vi "Set Cluster as Properties.vi"(8 "error in":errorcluster, 10 "Variant Cluster":variant, 11 "custom device ref in":T1 format="%.0x") -> (0 "error out":errorcluster, 3 "custom device ref out":T1 format="%.0x")   [LabVIEW 2020, in "AIM ARINC 664 Scripting.lvlib"]
uses:
  AIM ARINC 664 Scripting.lvlib
  <vilib>/NI VeriStand/Custom Device API/Custom Device Item Ref.ctl
  <vilib>/NI VeriStand/Custom Device API/Set Item Property (U32).vi
  <vilib>/NI VeriStand/Custom Device API/Set Item Property (Boolean).vi
  <vilib>/NI VeriStand/Custom Device API/Set Item Property (String).vi
  <vilib>/NI VeriStand/Custom Device API/Set Item Property (Path).vi
  <vilib>/NI VeriStand/Custom Device API/Custom Device API.lvlib
  <vilib>/Utility/Data Type/NI_Data Type.lvlib
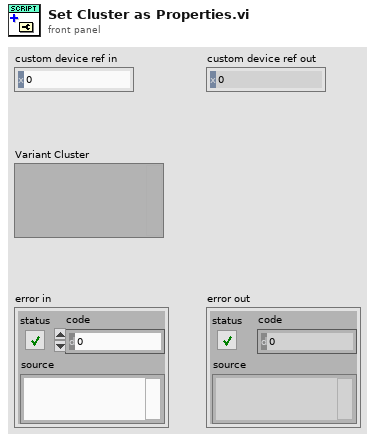
[diagram p1: front panel]
types:
  T1 = typedef "Custom Device API.lvlib/Custom Device Item Ref.ctl" = u64
  T2 = typedef "NI_Data Type.lvlib/Data Type.ctl" = enum8{"Invalid Type", "Void", "I8", "I16", "I32", "I64", "U8", "U16", "U32", "U64", "Single Float", "Double Float", "Extended Float", "Single Complex", "Double Complex", "Extended Complex", "Enum U8", "Enum U16", "Enum U32", "Enum U64", "Single Float With Unit", "Double Float With Unit", "Extended Float With Unit", "Single Complex with Unit", "Double Complex with Unit", "Extended Complex with Unit", "Boolean", "String", "Path", "Picture", "Tag", "Array", "Cluster", "Variant", "LV Variant", "Waveform", "Timestamp", "Digital Waveform", "Digital Data", "ExpressData", "Refnum", "External Data", "VI", "Poly VI", "LabVIEW Class Instance", "Fixed Point", "Set Collection", "Map Collection"}
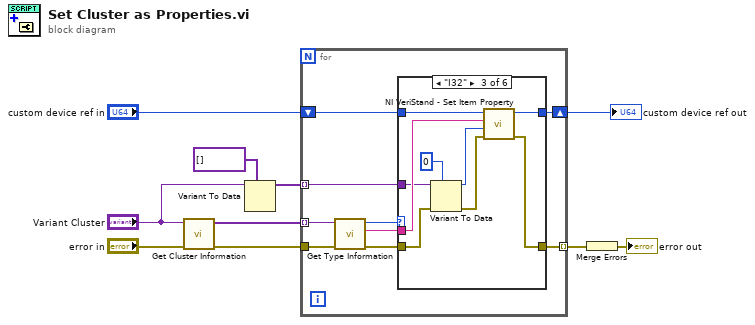
[diagram p0: block diagram]
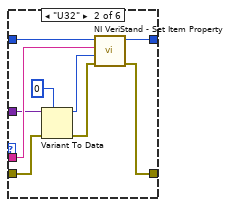
[diagram p3: hidden frame]
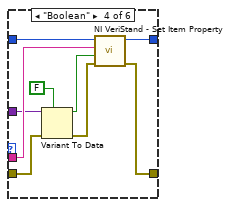
[diagram p4: hidden frame]
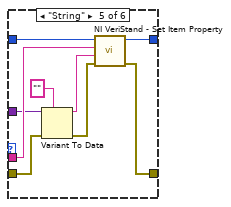
[diagram p5: hidden frame]
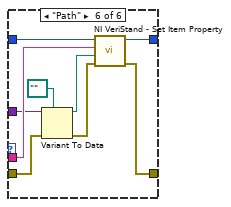
[diagram p6: hidden frame]
diagram:
  n1 = call <vilib>:"Get Cluster Information.vi"("error in (no error)"="error in", "variant"="Variant Cluster") -> ("error out"=w5:errorcluster, "cluster elements"=w6:variant[])  [unwired: 8 in]
  n2 = Variant To Data(type=variant[] [], Variant="Variant Cluster") -> (data=w4:variant[])  [unwired: 1 in, 1 out]
  n3 = for {
    tunnel: w6 -> [w19] mode=indexing
    shift-right: [w15] -> w8
    shift-left: "custom device ref in" -> [w16]
    tunnel: w4 -> [w11] mode=indexing
    tunnel: w5 -> [w18]
    tunnel: [w12] -> w9 mode=indexing
    n4 = call <vilib>:"Get Type Information.vi"("error in (no error)"=w18, "variant"=w19) -> ("error out"=w13:errorcluster, "name"=w17:string, "type"=w14:T2)  [unwired: 5 in, 2 out]
    n5 = case shown="\"I32\"" w14 {
      tunnel: w17 -> [_ w30 w39 w48 w57 w66]
      tunnel: w16 -> [w21 w29 w38 w47 w56 w65]
      tunnel: [w21 w28 w37 w46 w55 w64] -> w15
      tunnel: w13 -> [w20 w23 w32 w41 w50 w59]
      tunnel: [w20 w27 w36 w45 w54 w63] -> w12
      tunnel: w11 -> [_ w26 w35 w44 w53 w62]
      frame "Invalid Type", Default {
      }
      frame "U32" {
        n6 = Variant To Data(error in=w23, type=u32 0, Variant=w26) -> (data=w25:u32, error out=w22:errorcluster)
        n7 = call-poly <vilib>:"NI VeriStand - Set Item Property.vi"("error in (no error)"=w22, "Value"=w25, "Property Name"=w30, "Item Ref in"=w29) -> ("error out"=w27:errorcluster, "Item Ref out"=w28:T1)  [unwired: 5 in, 1 out]
      }
      frame "I32" {
        n8 = Variant To Data(error in=w32, type=0, Variant=w35) -> (data=w34:i32, error out=w31:errorcluster)
        n9 = call-poly <vilib>:"NI VeriStand - Set Item Property.vi"("error in (no error)"=w31, "Value"=w34, "Property Name"=w39, "Item Ref in"=w38) -> ("error out"=w36:errorcluster, "Item Ref out"=w37:T1)  [unwired: 5 in, 1 out]
      }
      frame "Boolean" {
        n10 = Variant To Data(error in=w41, type=FALSE, Variant=w44) -> (data=w43:bool, error out=w40:errorcluster)
        n11 = call-poly <vilib>:"NI VeriStand - Set Item Property.vi"("error in (no error)"=w40, "Value"=w43, "Property Name"=w48, "Item Ref in"=w47) -> ("error out"=w45:errorcluster, "Item Ref out"=w46:T1)  [unwired: 5 in, 1 out]
      }
      frame "String" {
        n12 = Variant To Data(error in=w50, type="", Variant=w53) -> (data=w52:string, error out=w49:errorcluster)
        n13 = call-poly <vilib>:"NI VeriStand - Set Item Property.vi"("error in (no error)"=w49, "Value"=w52, "Property Name"=w57, "Item Ref in"=w56) -> ("error out"=w54:errorcluster, "Item Ref out"=w55:T1)  [unwired: 5 in, 1 out]
      }
      frame "Path" {
        n14 = Variant To Data(error in=w59, type=path "", Variant=w62) -> (data=w61:path, error out=w58:errorcluster)
        n15 = call-poly <vilib>:"NI VeriStand - Set Item Property.vi"("error in (no error)"=w58, "Value"=w61, "Property Name"=w66, "Item Ref in"=w65) -> ("error out"=w63:errorcluster, "Item Ref out"=w64:T1)  [unwired: 5 in, 1 out]
      }
    }
  }
  "custom device ref out" <- w8
  n16 = Merge Errors(w9) -> (→"error out":errorcluster)
